vi "getTemperature.vi"(8 "error in (no error)":errorcluster, 11 "Pixelfly in":refnum<class "PixelflySA.lvclass">) -> (0 "error out":errorcluster, 2 "temperature":dbl, 3 "Pixelfly out":refnum<class "PixelflySA.lvclass">)   [LabVIEW 2009, in "PixelflySA.lvclass"]
uses:
  PixelflySA.lvclass
  PixelflySA.lvclass/PixelflySA.ctl
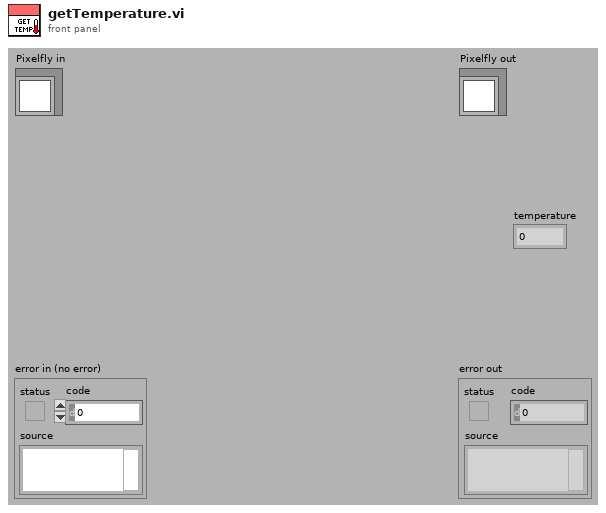
[diagram p1: front panel]
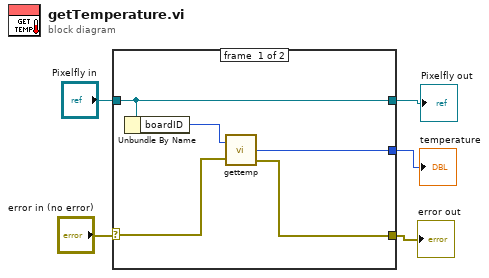
[diagram p0: block diagram]
diagram:
  n1 = case shown="No Error" "error in (no error)" {
    selector: "error in (no error)" -> [w6 w11]
    tunnel: "Pixelfly in" -> [w10 w12]
    tunnel: [w7 w11] -> w3
    tunnel: [w10 w12] -> w2
    tunnel: [w8 _] -> w1
    frame #0 {
      n2 = Unbundle By Name(w10) -> ("boardID"=w9:i32)
      n3 = call <instrlib>:"gettemp.vi"("Handle in"=w9, "error in (no error)"=w6) -> ("ccdtemp"=w8:i32, "error out"=w7:errorcluster)  [unwired: 1 out]
    }
    frame #1 {
    }
  }
  "error out" <- w3
  "Pixelfly out" <- w2
  "temperature" <- w1
